vi "manualDAQ_diag.vi"(6 "minimum value":dbl=-5.0 format="%0.2f", 7 "Rate":dbl, 8 "error in (no error)":errorcluster, 9 "Samples per Channel":i32, 10 "maximum value":dbl=5.0 format="%0.2f", 11 "physical channels":tag) -> (0 "error out":errorcluster, 3 "output waveform":waveform(dbl))   [LabVIEW 2013]
uses:
  <vilib>/DAQmx/read.llb/DAQmx Read (Analog 1D DBL 1Chan NSamp).vi
  <vilib>/DAQmx/create/channels.llb/DAQmx Create Channel (AI-Voltage-Basic).vi
  <vilib>/DAQmx/configure/timing.llb/DAQmx Timing (Sample Clock).vi
  <vilib>/DAQmx/miscellaneous.llb/DAQmx Fill In Error Info.vi
  <resource>/objmgr/daqmx.rc
panel:
  in  "input terminal configuration":i32(ring)=-1 items=["default"=-1, "RSE"=10083, "NRSE"=10078, "Differential"=10106, "Pseudodifferential"=12529]
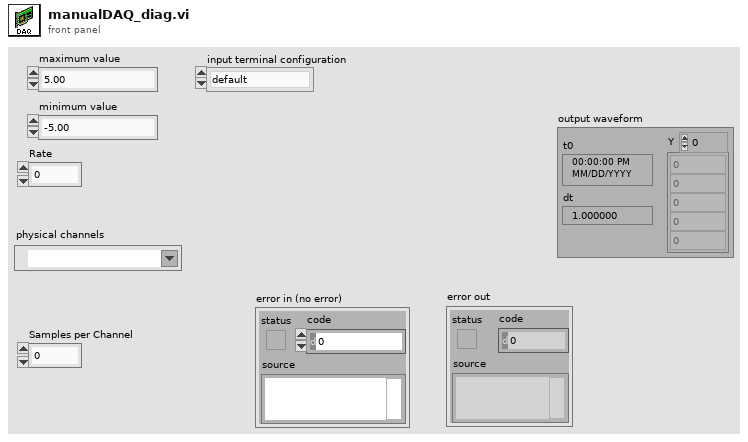
[diagram p1: front panel]
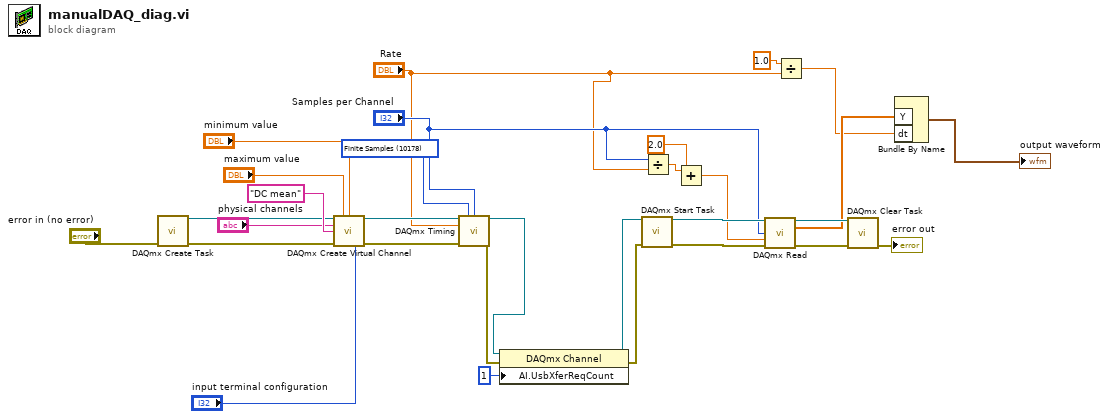
[diagram p0: block diagram]
diagram:
  w29 = 10178 items=["Finite Samples"=10178, "Continuous Samples"=10123] ("sample mode")
  n1 = call <vilib>:"DAQmx Create Task.vi"("error in"="error in (no error)") -> ("task out"=w7:refnum<k21>, "error out"=w8:errorcluster)  [unwired: 13 in]
  n2 = call-poly <vilib>:"DAQmx Create Virtual Channel.vi"("task in"=w7, "maximum value"="maximum value", "minimum value"="minimum value", "input terminal configuration"="input terminal configuration", "physical channels"="physical channels", "name to assign"="DC mean" ("new task name"), "error in"=w8) -> ("task out"=w18:refnum<k21>, "error out"=w19:errorcluster)  [unwired: 7 in]
  n3 = call-poly <vilib>:"DAQmx Timing.vi"("task/channels in"=w18, "sample mode"=w29, "samples per channel"="Samples per Channel", "rate"="Rate", "error in"=w19) -> ("task out"=w3:refnum<k21>, "error out"=w5:errorcluster)  [unwired: 9 in]
  n4 = property class="DAQmx Channel"(reference=w3, error in=w5, "AI.UsbXferReqCount"=u32 1) -> (reference out=w2:refnum<k21>, error out=w4:errorcluster)
  n5 = call <vilib>:"DAQmx Start Task.vi"("task/channels in"=w2, "error in"=w4) -> ("task out"=w27:refnum<k21>, "error out"=w25:errorcluster)  [unwired: 12 in]
  n6 = Divide(x="Samples per Channel", y="Rate") -> (x/y=w12:dbl)
  n7 = Add(x=w12, y=2.0) -> (x+y=w10:dbl)
  n8 = call-poly <vilib>:"DAQmx Read.vi"("task/channels in"=w27, "number of samples per channel"="Samples per Channel", "timeout"=w10, "error in"=w25) -> ("task out"=w28:refnum<k21>, "data"=w24:dbl[], "error out"=w30:errorcluster)  [unwired: 9 in]
  n9 = Divide(x=1.0, y="Rate") -> (x/y=w22:dbl)
  n10 = call <vilib>:"DAQmx Clear Task.vi"("task in"=w28, "error in"=w30) -> ("error out"=→"error out":errorcluster)  [unwired: 13 in]
  n11 = Bundle By Name("Y"=w24, "dt"=w22) -> (→"output waveform":waveform(dbl))  [unwired: 1 in]
